vi "Double FFT Mesurament RT (with BackNoise Remove) with Frequency Linearization Test.vi"() -> ()   [LabVIEW 2014]
uses:
  <vilib>/Platform/TimedLoop/XDataNode/timing_clust.ctl
  <vilib>/Platform/TimedLoop/XDataNode/nitl_modes.ctl
  <vilib>/Platform/TimedLoop/XDataNode/wakeup.ctl
  <vilib>/FPGAPlugInAG/sbRIO-9636/niLvFpga_Open_sbRIO-9636.vi
  <vilib>/rvi/interface/common/dynamic/niFpgaDynamicAddResources.vi
  <vilib>/Utility/error.llb/Error Cluster From Error Code.vi
  <vilib>/rvi/errors/niLvFpgaAdjustHostInterfaceError.vi
  <vilib>/rvi/interface/common/niFpgaWaitOnOcc.vi
  <vilib>/FPGAPlugInAG/Dynamic/niLvFpga_Run_Dynamic.vi
  <vilib>/FPGAPlugInAG/Dynamic/niLvFpga_Abort_Dynamic.vi
  <vilib>/FPGAPlugInAG/Dynamic/niLvFpga_Reset_Dynamic.vi
  <vilib>/FPGAPlugInAG/Dynamic/niLvFpga_Close_Dynamic.vi
  <vilib>/rvi/interface/nirviOpenFPGA/nirviOpenFPGA.xnode
  FPGA Bitfiles/LaserDistanceSen_FPGATarget_DoubleFFTMesuram_6dDziXQAIGE.lvbitx
  FPGA Target/Test VIs/Double FFT Mesurament Test with Background Noise Remove.vi
  <vilib>/rvi/interface/nirviReadWriteControl/nirviReadWriteControl.xnode
  <vilib>/rvi/interface/nirviMethod/nirviMethod.xnode
  <vilib>/Platform/TimedLoop/XDataNode/XDataNode.xnode
  <vilib>/rvi/interface/nirviCloseFPGA/nirviCloseFPGA.xnode
  <vilib>/FPGAPlugInAG/Dynamic/niLvFpga_ConfigureFifo_Dynamic.vi
  <vilib>/rvi/errors/niLvFpgaMergeErrorWithErrorCode.vi
  <vilib>/FPGAPlugInAG/Dynamic/niLvFpga_StartFifo_Dynamic.vi
  <vilib>/rvi/interface/Simulation/niFpgaSimulationCallBeginRW.vi
  <vilib>/FPGAPlugInAG/Dynamic/niLvFpga_ReadFifo_Dynamic.vi
  <vilib>/Platform/TimedLoop/XDataNode/XDNodeRunTimeDep.lvlib
  NiFpgaLv.dll
panel:
  in  "SubtractionType":T1(ring)
  out "Fondo Signal":dbl[](graph)
  in  "nbit":i32=7
  in  "LowPass Filter: Low cutoff frequency":dbl=20000.0 format="%#_13g"
  in  "PolyFitting: Poly Grade":dbl=5.0
  in  "Scale Factor Rising":dbl=0.5
  out "2) Std Dev":dbl
  out "1) Std Dev":dbl
  in  "Scale Factor Falling":dbl=0.5
  in  "Triangolo dritto":bool=TRUE
  in  "Acrive  Smooth":bool
  out "Complete SkewTri":dbl[](graph)
  out "2) Tri edge RISING":dbl[](graph)
  out "1) Tri edge FALLING":dbl[](graph)
  out "1) Ext Mean Time Curve":dbl[](graph)
  out "2) Ext Mean Time Curve":dbl[](graph)
  out "2) Mean Freq Curve Rising":dbl[](graph)
  out "1) Mean Freq Curve Falling":dbl[](graph)
  out "2) Freq curve":dbl[](graph)
  out "1) Freq curve":dbl[](graph)
  in  "FFT Sliding Win Size":i32=128
  out "1) SmoothSubSig":dbl[](graph)
  out "2) SmoothSubSig":dbl[](graph)
  in  "Acrive Fit":bool=TRUE
  in  "Poly Order":i32=3
  in  "Side points":i32=13
  in  "Poly Grade":dbl=5.0
  out "2) Signal&Fit 2":dbl[][](graph)
  out "1) Signal&Fit":dbl[][](graph)
  in  "tieni premuto per":i32=1
  out "Current Sig lin":i32
  in  "Acrive Linearization":bool
  in  "# Measurements for Linearization":i32=10
  in  "?":bool
  out "maxbin_secondFFT":i32
  out "maxbin_firstFFT":i32
  out "f_rise":dbl
  out "f_fall":dbl
  out "f_mean":dbl
  out "Velocity (m/s)":dbl
  out "Distance (m)":dbl
  in  "Initial Latency points":u32(slide) scale=0.0..1249.0
  out "Second FFT (bin)":dbl[](graph)
  out "Second Signal (points) - Rising Triangular":dbl[](graph)
  out "First FFT (bin)":dbl[](graph)
  out "First Signal (points) - Falling Triangular":dbl[](graph)
  in  "Snapshot":bool
  in  "Windowing":T2(ring)
  in  "first bin":i32=5
  in  "last bin":i32=255
  in  "lower limit 2":u32(slide)=738 scale=625.0..738.0
  in  "lower limit 1":u32(slide)=113 scale=0.0..113.0
  # "Fondo pre-elaborato"
  # "WARNING:\nOnce pressed wait untill the end of operation"
  # "OFFLINE parameters"
  # "Triangolo storto\nda costante"
  # "Max Detection FFT bin range"
  # "ONLINE parameters"
  # "Se la sottrazione del fondo non è eseguita su FPGA.\n Attivarla per eseguirla lato RT"
  # "Smoothing (S-G Params)"
  # "Fitting"
  # "ONLY POWER OF 2"
  # "Min: 2 Max: 256 (2, 4, 8, 16, 32, 64, 128, 256)"
  # "LINEARIZATION FINAL RESULTS"
  # "dev standard (max-min)"
  # "%"
  # "%"
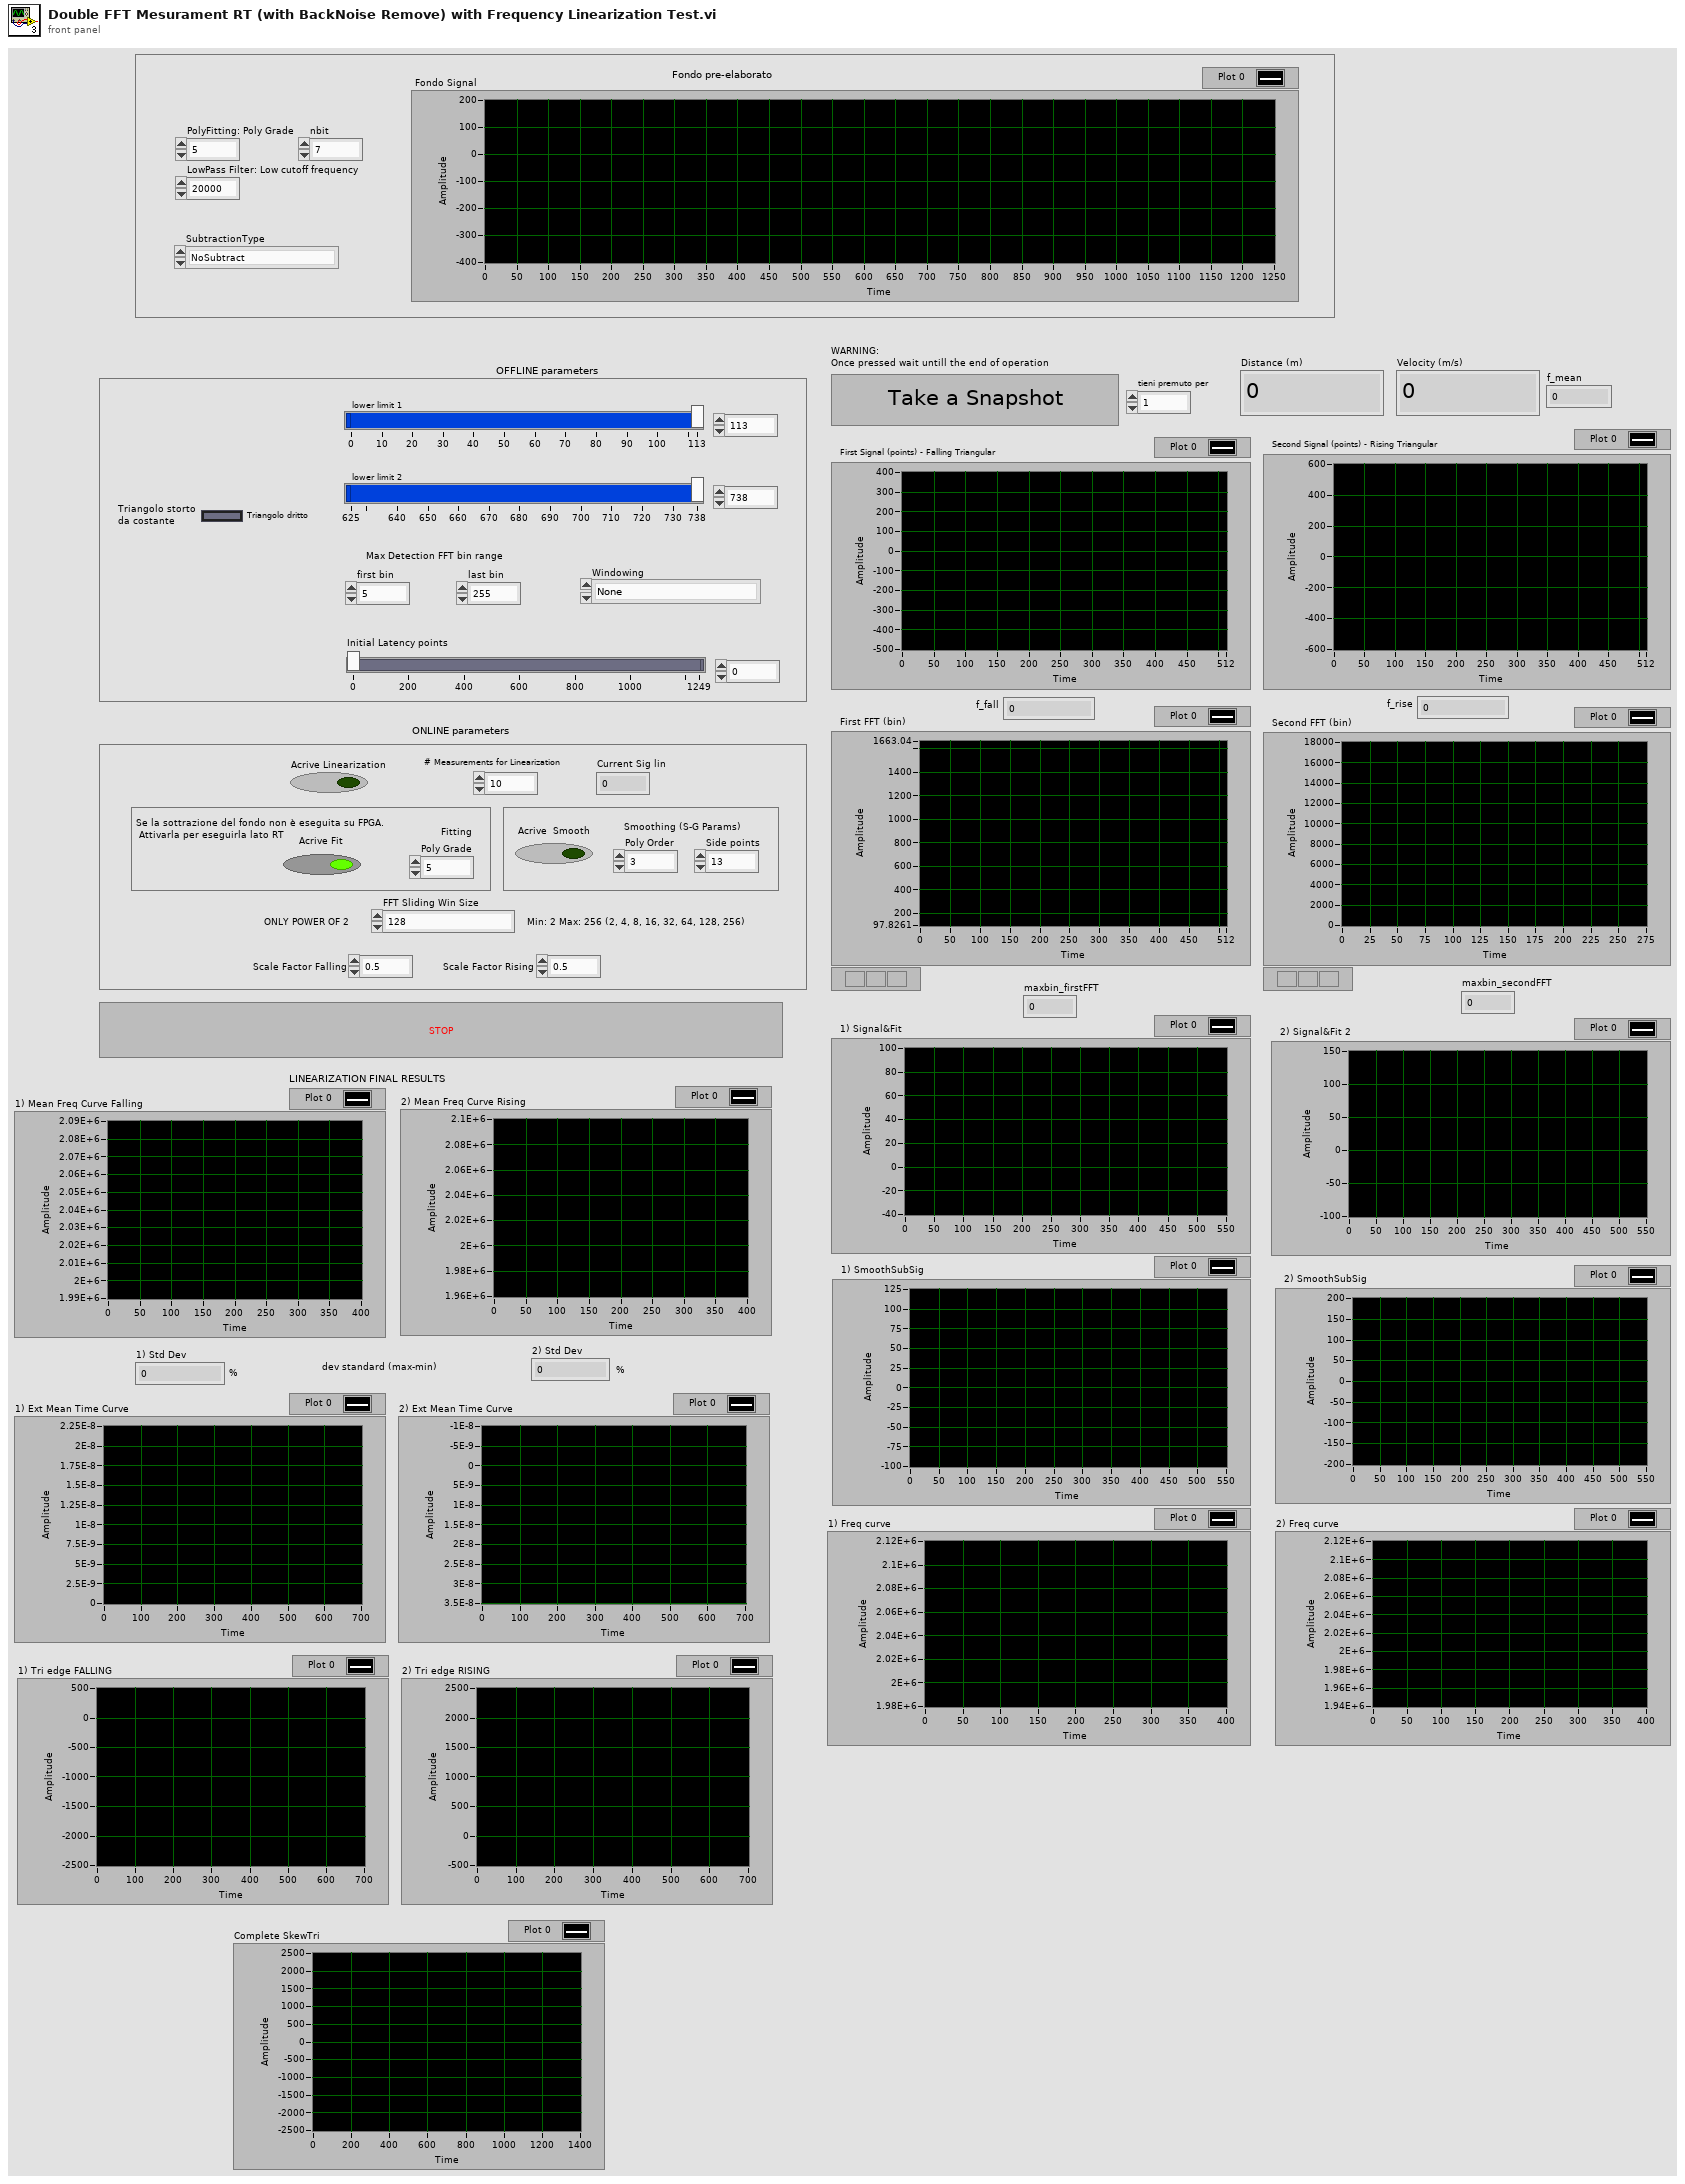
[diagram p1: front panel]
types:
  T1 = enum16{"NoSubtract", "StartingCurve", "LowPass", "PolyFitting"}
  T2 = enum16{"None", "Hanning", "Hamming", "Blackman", "Blackman-Harris"}
  T3 = typedef "XDNodeRunTimeDep.lvlib/timing_clust.ctl" = cluster{"Expected End [f-1]":u64, "Actual End [f-1]":u64, "Finished Late? [f-1]":bool, "Expected End [i-1]":u64, "Actual End [i-1]":u64, "Finished Late? [i-1]":bool, "Expected Start [i]":u64, "Actual Start [i]":u64, "Expected Start [f]":u64, "Actual Start [f]":u64, "Source Name":string, "Structure Name":string, "Period":i64, "Deadline":i64, "Offset":i64, "Start":i64, "Priority":i32, "Timeout":i32, "Mode":T4, "Wakeup Reason":T5, "Error":errorcluster, "Source Type":string, "Secondary Source Type":string, "Global End Time":u64, "Global Start Time":u64, "Frame Duration":u64, "Iteration Duration":u64, "Assigned CPU":i32, "I/O Scan Engine Mode":u32}
  T4 = typedef "XDNodeRunTimeDep.lvlib/nitl_modes.ctl" = enum32{"No Change", "Process missed periods, maintain original phase", "Discard missed periods, maintain original phase", "Process missed periods, ignore original phase", "Discard missed periods, ignore original phase"}
  T5 = typedef "XDNodeRunTimeDep.lvlib/wakeup.ctl" = enum32{"Normal", "Aborted", "Asynchronous wakeup", "Timing source error", "Timed loop error", "Timeout"}
  T6 = typedef "NI_Matrix.lvlib/RealMatrix.ctl" = dbl[][]
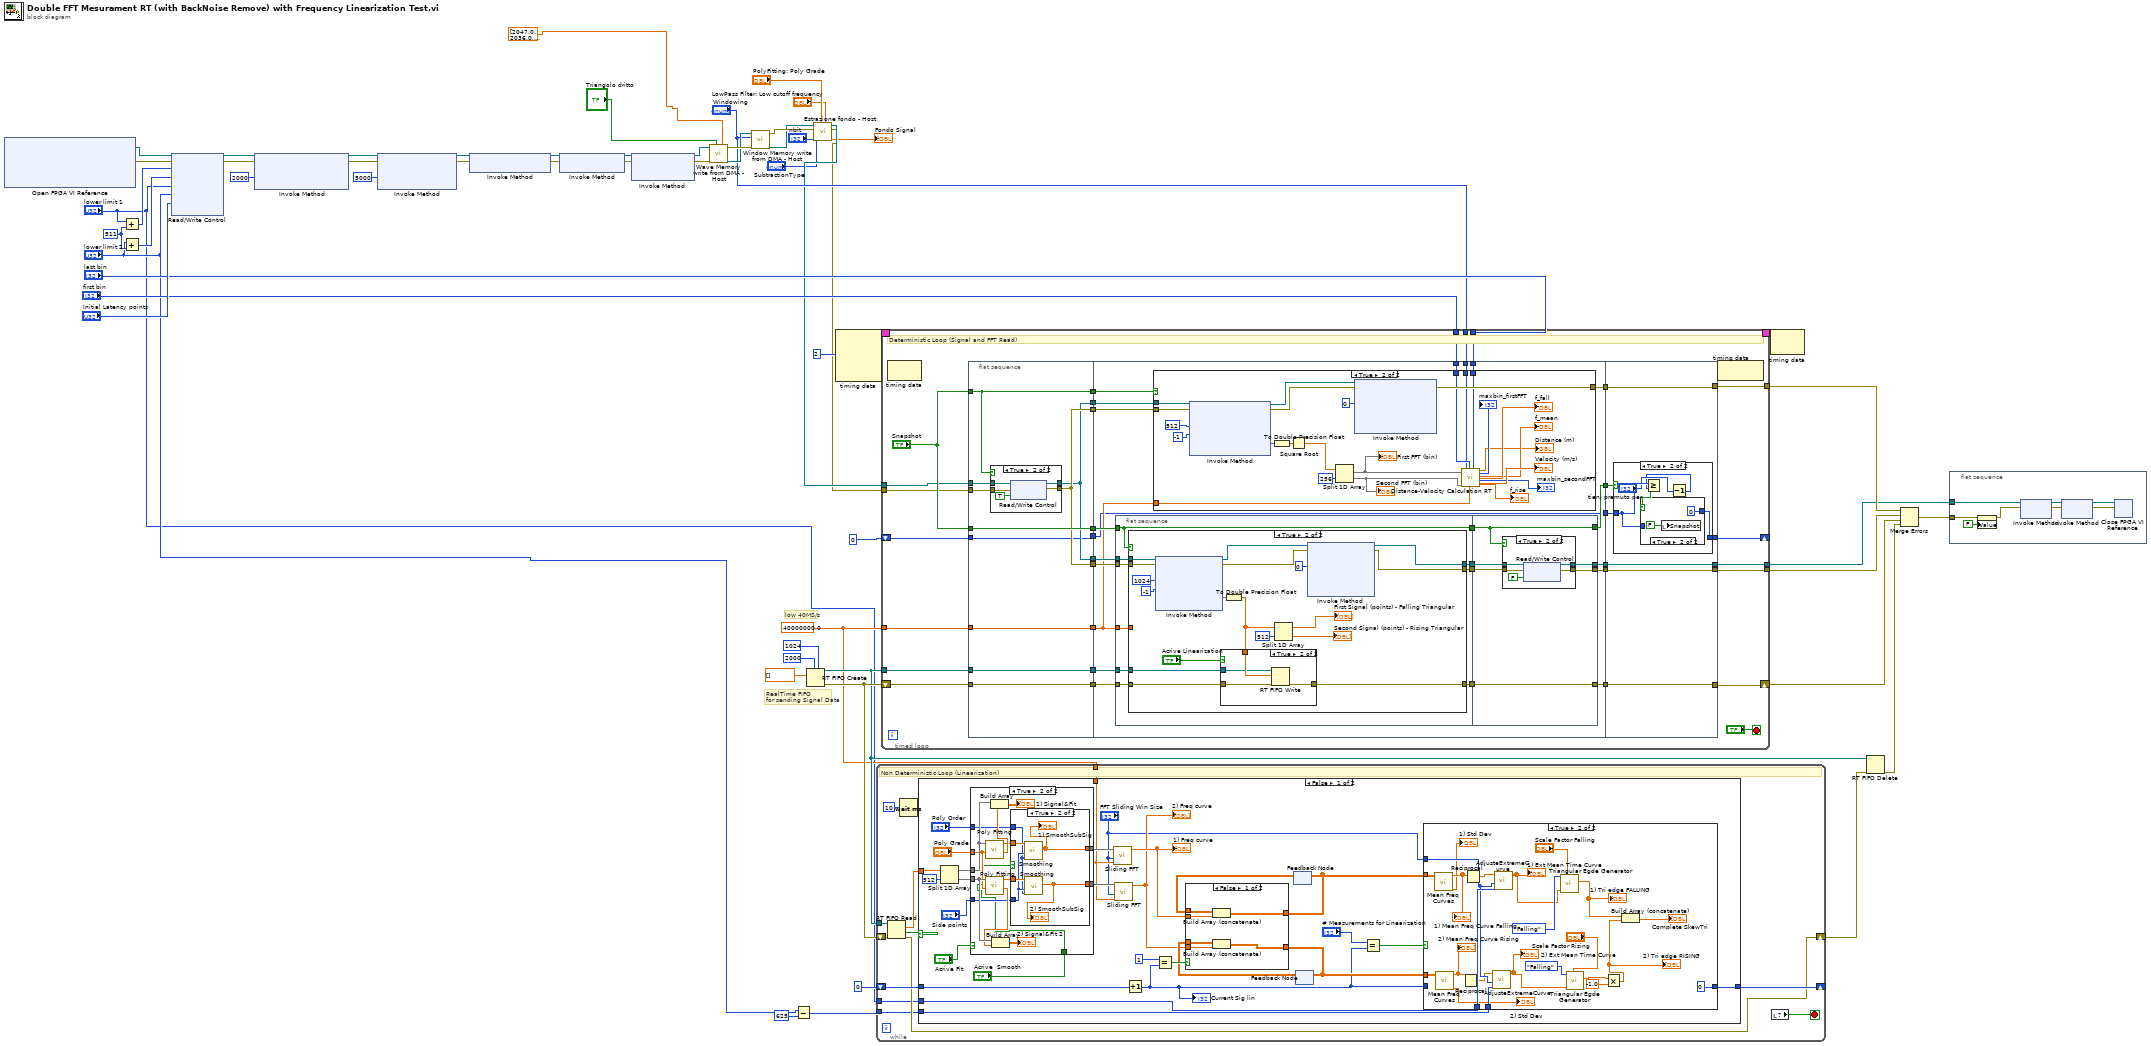
[diagram p0: block diagram]
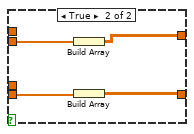
[diagram p5: hidden frame]
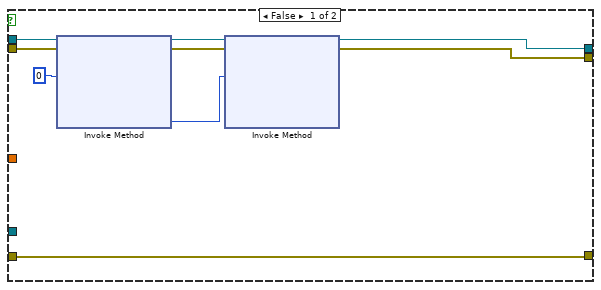
[diagram p8: hidden frame]
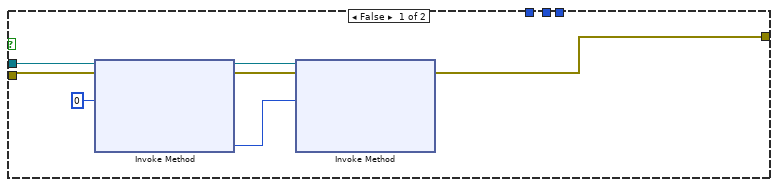
[diagram p11: hidden frame]
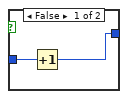
[diagram p13: hidden frame]
diagram:
  w56 = u32 511 ("y")
  w13 = 40000000.0 ("Sample Rate (S/s)")
  # "RealTime FIFO \nfor sending Signal Data"
  # "low 40MS/s"
  n1 = xnode "Open FPGA VI Reference"() -> ("FPGA VI Reference Out"=w55:refnum<k20>, "error out"=w54:errorcluster)  [unwired: 2 in]
  n2 = Add(x="lower limit 1", y=w56) -> (x+y=w58:u32)
  n3 = Add(x="lower limit 2", y=w56) -> (x+y=w57:u32)
  n4 = xnode "Read/Write Control"("FPGA VI Reference In"=w55, "error in"=w54, "upper limit 1"=w58, "upper limit 2"=w57, "lower limit 1"="lower limit 1", "lower limit 2"="lower limit 2", "Latency points"="Initial Latency points") -> ("FPGA VI Reference Out"=w53:refnum<k20>, "error out"=w52:errorcluster)  [unwired: 1 in]
  n5 = xnode "Invoke Method"("FPGA VI Reference In"=w53, "error in"=w52, "Requested Depth"=u32 2000) -> ("FPGA VI Reference Out"=w31:refnum<k20>, "error out"=w32:errorcluster)  [unwired: 1 out]
  n6 = xnode "Invoke Method"("FPGA VI Reference In"=w31, "error in"=w32, "Requested Depth"=u32 5000) -> ("FPGA VI Reference Out"=w45:refnum<k20>, "error out"=w46:errorcluster)  [unwired: 1 out]
  n7 = xnode "Invoke Method"("FPGA VI Reference In"=w45, "error in"=w46) -> ("FPGA VI Reference Out"=w29:refnum<k20>, "error out"=w30:errorcluster)
  n8 = xnode "Invoke Method"("FPGA VI Reference In"=w29, "error in"=w30) -> ("FPGA VI Reference Out"=w43:refnum<k20>, "error out"=w44:errorcluster)
  n9 = xnode "Invoke Method"("FPGA VI Reference In"=w43, "error in"=w44) -> ("FPGA VI Reference Out"=w49:refnum<k20>, "error out"=w48:errorcluster)  [unwired: 1 in]
  n10 = call "Wave Memory write from DMA - Host.vi"("Custom Triangular Signal (fal-ris)"=dbl[] [2047.0, 2036.0, 2024.0, 2013.0, 2002.0, 1990.0, 1979.0, 1968.0, 1956.0, 1945.0, 1934.0, 1923.0, 1912.0, 1900.0, 1889.0, 1878.0, 1867.0, 1856.0, 1845.0, 1833.0, 1822.0, 1811.0, 1800.0, 1789.0, 1778.0, 1767.0, 1756.0, 1745.0, 1734.0, 1723.0, 1712.0, 1702.0, 1691.0, 1680.0, 1669.0, 1658.0, 1647.0, 1636.0, 1626.0, 1615.0, 1604.0, 1593.0, 1583.0, 1572.0, 1561.0, 1550.0, 1540.0, 1529.0, 1518.0, 1508.0, 1497.0, 1487.0, 1476.0, 1465.0, 1455.0, 1444.0, 1434.0, 1423.0, 1413.0, 1402.0, 1392.0, 1381.0, 1371.0, 1360.0, 1350.0, 1340.0, 1329.0, 1319.0, 1309.0, 1298.0, 1288.0, 1278.0, 1267.0, 1257.0, 1247.0, 1237.0, 1226.0, 1216.0, 1206.0, 1196.0, 1186.0, 1176.0, 1165.0, 1155.0, 1145.0, 1135.0, 1125.0, 1115.0, 1105.0, 1095.0, 1085.0, 1075.0, 1065.0, 1055.0, 1045.0, 1035.0, 1025.0, 1015.0, 1006.0, 996.0, 986.0, 976.0, 966.0, 956.0, 947.0, 937.0, 927.0, 917.0, 908.0, 898.0, 888.0, 879.0, 869.0, 859.0, 850.0, 837.0, 826.0, 816.0, 804.0, 796.0, 788.0, 778.0, 769.0, 758.0, 750.0, 743.0, 733.0, 724.0, 717.0, 709.0, 701.0, 693.0, 686.0, 677.0, 669.0, 661.0, 653.0, 645.0, 638.0, 630.0, 622.0, 615.0, 607.0, 599.0, 592.0, 583.0, 576.0, 569.0, 561.0, 554.0, 547.0, 539.0, 532.0, 525.0, 518.0, 509.0, 501.0, 492.0, 486.0, 478.0, 471.0, 463.0, 456.0, 450.0, 442.0, 435.0, 429.0, 421.0, 415.0, 408.0, 401.0, 394.0, 388.0, 381.0, 375.0, 368.0, 361.0, 355.0, 349.0, 342.0, 336.0, 330.0, 323.0, 317.0, 311.0, 304.0, 298.0, 292.0, 286.0, 279.0, 273.0, 267.0, 261.0, 255.0, 249.0, 242.0, 236.0, 230.0, 224.0, 218.0, 212.0, 206.0, 200.0, 194.0, 187.0, 181.0, 175.0, 169.0, 163.0, 157.0, 150.0, 144.0, 138.0, 132.0, 125.0, 119.0, 113.0, 107.0, 101.0, 95.0, 88.0, 82.0, 77.0, 71.0, 65.0, 59.0, 53.0, 47.0, 41.0, 35.0, 29.0, 23.0, 18.0, 11.0, 6.0, 0.0, -6.0, -12.0, -18.0, -23.0, -29.0, -35.0, -41.0, -47.0, -52.0, -58.0, -64.0, -69.0, -75.0, -81.0, -87.0, -92.0, -98.0, -104.0, -109.0, -115.0, -121.0, -126.0, -132.0, -138.0, -144.0, -149.0, -155.0, -161.0, -166.0, -172.0, -177.0, -183.0, -189.0, -194.0, -200.0, -205.0, -211.0, -216.0, -222.0, -227.0, -233.0, -238.0, -244.0, -249.0, -255.0, -260.0, -266.0, -271.0, -277.0, -283.0, -288.0, -294.0, -299.0, -304.0, -310.0, -315.0, -321.0, -326.0, -331.0, -337.0, -342.0, -348.0, -353.0, -358.0, -364.0, -369.0, -375.0, -380.0, -385.0, -391.0, -396.0, -402.0, -407.0, -413.0, -418.0, -423.0, -429.0, -434.0, -439.0, -445.0, -450.0, -456.0, -461.0, -466.0, -472.0, -477.0, -483.0, -488.0, -493.0, -499.0, -504.0, -510.0, -515.0, -520.0, -526.0, -531.0, -537.0, -542.0, -548.0, -553.0, -558.0, -564.0, -569.0, -574.0, -580.0, -585.0, -590.0, -596.0, -601.0, -606.0, -612.0, -617.0, -622.0, -628.0, -633.0, -638.0, -644.0, -649.0, -654.0, -660.0, -665.0, -670.0, -676.0, -681.0, -686.0, -692.0, -697.0, -702.0, -708.0, -713.0, -718.0, -723.0, -729.0, -734.0, -739.0, -744.0, -750.0, -755.0, -760.0, -765.0, -771.0, -776.0, -781.0, -786.0, -792.0, -797.0, -802.0, -807.0, -812.0, -818.0, -823.0, -828.0, -833.0, -839.0, -844.0, -849.0, -854.0, -859.0, -865.0, -870.0, -875.0, -880.0, -885.0, -891.0, -896.0, -901.0, -906.0, -911.0, -916.0, -922.0, -927.0, -932.0, -937.0, -943.0, -948.0, -953.0, -958.0, -963.0, -969.0, -974.0, -979.0, -984.0, -989.0, -995.0, -1000.0, -1005.0, -1010.0, -1015.0, -1021.0, -1026.0, -1031.0, -1036.0, -1041.0, -1047.0, -1052.0, -1057.0, -1062.0, -1067.0, -1073.0, -1078.0, -1083.0, -1088.0, -1093.0, -1099.0, -1104.0, -1109.0, -1114.0, -1119.0, -1124.0, -1130.0, -1135.0, -1140.0, -1145.0, -1150.0, -1156.0, -1161.0, -1166.0, -1171.0, -1176.0, -1182.0, -1187.0, -1192.0, -1197.0, -1202.0, -1207.0, -1213.0, -1218.0, -1223.0, -1228.0, -1233.0, -1238.0, -1244.0, -1249.0, -1254.0, -1259.0, -1264.0, -1269.0, -1275.0, -1280.0, -1285.0, -1290.0, -1295.0, -1300.0, -1305.0, -1311.0, -1316.0, -1321.0, -1326.0, -1331.0, -1336.0, -1342.0, -1347.0, -1352.0, -1357.0, -1362.0, -1367.0, -1372.0, -1378.0, -1383.0, -1388.0, -1393.0, -1398.0, -1403.0, -1408.0, -1414.0, -1419.0, -1424.0, -1429.0, -1434.0, -1439.0, -1444.0, -1450.0, -1455.0, -1460.0, -1465.0, -1470.0, -1475.0, -1480.0, -1486.0, -1491.0, -1496.0, -1501.0, -1506.0, -1511.0, -1516.0, -1522.0, -1527.0, -1532.0, -1537.0, -1542.0, -1547.0, -1552.0, -1558.0, -1563.0, -1568.0, -1573.0, -1578.0, -1583.0, -1588.0, -1593.0, -1599.0, -1604.0, -1609.0, -1614.0, -1619.0, -1624.0, -1629.0, -1634.0, -1640.0, -1645.0, -1650.0, -1655.0, -1660.0, -1665.0, -1670.0, -1675.0, -1681.0, -1686.0, -1691.0, -1696.0, -1701.0, -1706.0, -1711.0, -1716.0, -1722.0, -1727.0, -1732.0, -1737.0, -1742.0, -1747.0, -1752.0, -1757.0, -1762.0, -1768.0, -1773.0, -1778.0, -1783.0, -1788.0, -1793.0, -1798.0, -1803.0, -1808.0, -1814.0, -1819.0, -1824.0, -1829.0, -1834.0, -1839.0, -1844.0, -1849.0, -1854.0, -1859.0, -1865.0, -1870.0, -1875.0, -1880.0, -1885.0, -1890.0, -1895.0, -1900.0, -1905.0, -1911.0, -1916.0, -1921.0, -1926.0, -1931.0, -1936.0, -1941.0, -1946.0, -1951.0, -1956.0, -1961.0, -1967.0, -1972.0, -1977.0, -1982.0, -1987.0, -1992.0, -1997.0, -2002.0, -2007.0, -2012.0, -2017.0, -2023.0, -2028.0, -2033.0, -2038.0, -2043.0, -2048.0, -2047.0, -2034.0, -2021.0, -2009.0, -1996.0, -1983.0, -1970.0, -1957.0, -1945.0, -1932.0, -1919.0, -1907.0, -1894.0, -1881.0, -1869.0, -1856.0, -1844.0, -1831.0, -1819.0, -1806.0, -1794.0, -1781.0, -1769.0, -1757.0, -1744.0, -1732.0, -1719.0, -1707.0, -1695.0, -1682.0, -1670.0, -1658.0, -1646.0, -1634.0, -1621.0, -1609.0, -1597.0, -1585.0, -1573.0, -1561.0, -1549.0, -1537.0, -1525.0, -1513.0, -1501.0, -1489.0, -1477.0, -1465.0, -1453.0, -1441.0, -1429.0, -1417.0, -1405.0, -1394.0, -1382.0, -1370.0, -1358.0, -1347.0, -1335.0, -1323.0, -1312.0, -1300.0, -1288.0, -1277.0, -1265.0, -1254.0, -1242.0, -1231.0, -1219.0, -1208.0, -1196.0, -1185.0, -1173.0, -1162.0, -1150.0, -1139.0, -1128.0, -1116.0, -1105.0, -1094.0, -1083.0, -1071.0, -1060.0, -1049.0, -1038.0, -1027.0, -1015.0, -1004.0, -993.0, -982.0, -971.0, -960.0, -949.0, -938.0, -927.0, -916.0, -905.0, -894.0, -883.0, -873.0, -862.0, -851.0, -840.0, -829.0, -819.0, -808.0, -797.0, -786.0, -776.0, -765.0, -754.0, -744.0, -733.0, -722.0, -712.0, -697.0, -685.0, -674.0, -661.0, -652.0, -643.0, -632.0, -622.0, -610.0, -602.0, -594.0, -583.0, -574.0, -566.0, -558.0, -550.0, -542.0, -534.0, -525.0, -516.0, -507.0, -499.0, -491.0, -483.0, -475.0, -467.0, -459.0, -451.0, -443.0, -435.0, -426.0, -419.0, -411.0, -404.0, -396.0, -388.0, -381.0, -373.0, -366.0, -359.0, -349.0, -341.0, -331.0, -325.0, -317.0, -309.0, -301.0, -295.0, -288.0, -280.0, -273.0, -266.0, -259.0, -252.0, -246.0, -239.0, -231.0, -225.0, -219.0, -212.0, -205.0, -199.0, -192.0, -186.0, -180.0, -173.0, -167.0, -161.0, -155.0, -148.0, -142.0, -136.0, -130.0, -124.0, -118.0, -112.0, -106.0, -100.0, -94.0, -88.0, -82.0, -76.0, -70.0, -64.0, -58.0, -52.0, -46.0, -40.0, -34.0, -28.0, -21.0, -15.0, -9.0, -3.0, 2.0, 9.0, 15.0, 21.0, 27.0, 33.0, 39.0, 45.0, 51.0, 57.0, 63.0, 69.0, 75.0, 81.0, 86.0, 92.0, 98.0, 103.0, 110.0, 116.0, 121.0, 127.0, 133.0, 138.0, 144.0, 149.0, 155.0, 161.0, 166.0, 172.0, 177.0, 183.0, 189.0, 194.0, 200.0, 205.0, 211.0, 216.0, 221.0, 227.0, 232.0, 238.0, 243.0, 249.0, 254.0, 259.0, 265.0, 270.0, 276.0, 281.0, 286.0, 292.0, 297.0, 303.0, 308.0, 314.0, 319.0, 324.0, 329.0, 335.0, 340.0, 345.0, 351.0, 356.0, 361.0, 366.0, 371.0, 377.0, 382.0, 387.0, 392.0, 397.0, 403.0, 408.0, 413.0, 418.0, 423.0, 429.0, 434.0, 439.0, 444.0, 449.0, 454.0, 459.0, 464.0, 469.0, 474.0, 479.0, 484.0, 489.0, 494.0, 499.0, 504.0, 509.0, 514.0, 520.0, 525.0, 530.0, 535.0, 540.0, 545.0, 550.0, 555.0, 560.0, 565.0, 570.0, 575.0, 580.0, 585.0, 590.0, 595.0, 600.0, 605.0, 610.0, 615.0, 620.0, 625.0, 630.0, 636.0, 641.0, 646.0, 651.0, 656.0, 661.0, 666.0, 671.0, 676.0, 681.0, 686.0, 691.0, 696.0, 701.0, 706.0, 711.0, 716.0, 721.0, 726.0, 731.0, 736.0, 741.0, 746.0, 751.0, 756.0, 761.0, 765.0, 770.0, 775.0, 780.0, 785.0, 790.0, 795.0, 800.0, 805.0, 810.0, 815.0, 820.0, 825.0, 829.0, 834.0, 839.0, 844.0, 849.0, 854.0, 859.0, 864.0, 868.0, 873.0, 878.0, 883.0, 888.0, 893.0, 897.0, 902.0, 907.0, 912.0, 917.0, 921.0, 926.0, 931.0, 936.0, 941.0, 945.0, 950.0, 955.0, 960.0, 965.0, 969.0, 974.0, 979.0, 984.0, 988.0, 993.0, 998.0, 1003.0, 1007.0, 1012.0, 1017.0, 1022.0, 1027.0, 1031.0, 1036.0, 1041.0, 1046.0, 1051.0, 1055.0, 1060.0, 1065.0, 1070.0, 1075.0, 1079.0, 1084.0, 1089.0, 1094.0, 1098.0, 1103.0, 1108.0, 1113.0, 1118.0, 1122.0, 1127.0, 1132.0, 1137.0, 1141.0, 1146.0, 1151.0, 1156.0, 1161.0, 1165.0, 1170.0, 1175.0, 1180.0, 1184.0, 1189.0, 1194.0, 1199.0, 1204.0, 1208.0, 1213.0, 1218.0, 1223.0, 1227.0, 1232.0, 1237.0, 1242.0, 1246.0, 1251.0, 1256.0, 1261.0, 1265.0, 1270.0, 1275.0, 1280.0, 1284.0, 1289.0, 1294.0, 1299.0, 1303.0, 1308.0, 1313.0, 1318.0, 1322.0, 1327.0, 1332.0, 1336.0, 1341.0, 1346.0, 1351.0, 1355.0, 1360.0, 1365.0, 1370.0, 1374.0, 1379.0, 1384.0, 1388.0, 1393.0, 1398.0, 1403.0, 1407.0, 1412.0, 1417.0, 1421.0, 1426.0, 1431.0, 1436.0, 1440.0, 1445.0, 1450.0, 1454.0, 1459.0, 1464.0, 1469.0, 1473.0, 1478.0, 1483.0, 1487.0, 1492.0, 1497.0, 1502.0, 1506.0, 1511.0, 1516.0, 1520.0, 1525.0, 1530.0, 1535.0, 1539.0, 1544.0, 1549.0, 1553.0, 1558.0, 1563.0, 1567.0, 1572.0, 1577.0, 1582.0, 1586.0, 1591.0, 1596.0, 1600.0, 1605.0, 1610.0, 1614.0, 1619.0, 1624.0, 1628.0, 1633.0, 1638.0, 1643.0, 1647.0, 1652.0, 1657.0, 1661.0, 1666.0, 1671.0, 1675.0, 1680.0, 1685.0, 1689.0, 1694.0, 1699.0, 1703.0, 1708.0, 1713.0, 1717.0, 1722.0, 1727.0, 1731.0, 1736.0, 1741.0, 1746.0, 1750.0, 1755.0, 1760.0, 1764.0, 1769.0, 1774.0, 1778.0, 1783.0, 1788.0, 1792.0, 1797.0, 1802.0, 1806.0, 1811.0, 1816.0, 1820.0, 1825.0, 1830.0, 1834.0, 1839.0, 1844.0, 1848.0, 1853.0, 1858.0, 1862.0, 1867.0, 1871.0, 1876.0, 1881.0, 1885.0, 1890.0, 1895.0, 1899.0, 1904.0, 1909.0, 1913.0, 1918.0, 1923.0, 1927.0, 1932.0, 1937.0, 1941.0, 1946.0, 1951.0, 1955.0, 1960.0, 1965.0, 1969.0, 1974.0, 1978.0, 1983.0, 1988.0, 1992.0, 1997.0, 2002.0, 2006.0, 2011.0, 2016.0, 2020.0, 2025.0, 2029.0, 2034.0, 2039.0, 2043.0, 2048.0] ("Complete SkewTri"), "Triangolo dritto?"="Triangolo dritto", "error in"=w48, "FPGA VI Reference In"=w49) -> ("FPGA VI Reference Out"=w34:refnum<k20>, "error out"=w47:errorcluster)  [unwired: 5 in, 1 out]
  n11 = call "Window Memory write from DMA - Host.vi"("error in"=w47, "Enum"="Windowing", "FPGA VI Reference In"=w34) -> ("FPGA VI Reference Out"=w8:refnum<k20>, "error out"=w9:errorcluster)  [unwired: 5 in, 2 out]
  n12 = Subtract(x="lower limit 2", y=u32 625) -> (x-y=w15:u32)
  n13 = RT FIFO Create(1:dbl[] [] ("double precision float"), 4:u32 2000 ("size (10)"), 6:u32 1024 ("elements in array (1)")) -> (8:w21:refnum<k33>, 11:w23:errorcluster)  [unwired: 5 in, 1 out]
  n14 = call "Estrazione fondo - Host.vi"("LowPass Filter: Low cutoff frequency"="LowPass Filter: Low cutoff frequency", "PolyFitting: Poly Grade"="PolyFitting: Poly Grade", "nbit"="nbit", "SubtractionType"="SubtractionType", "error in"=w9, "FPGA VI Reference In"=w8) -> ("Fondo Signal"=→"Fondo Signal":dbl[], "error out"=w6:errorcluster, "FPGA VI Reference Out"=w7:refnum<k20>)  [unwired: 2 in, 1 out]
  n15 = node-c288(i64 2 ("Period")) -> (w42:T3)  [unwired: 3 in]
  n16 = while {
    shift-right: [w62] -> w20
    shift-left: w23 -> [w64]
    tunnel: w21 -> [w69]
    shift-right: [w63] -> _
    shift-left: 0 -> [w67]
    tunnel: "lower limit 1" -> [w59]
    tunnel: w15 -> [w60]
    tunnel: w13 -> [w61]
    stop <- w68 stop-if-true
    # "Non Deterministic Loop (Linearization)"
    n17 = RT FIFO Read(0:w69, 3:w64) -> (9:w66:dbl[], 10:w65:bool, 11:w62:errorcluster)  [unwired: 2 in, 2 out]
    n18 = Wait (ms)(milliseconds to wait=u32 10 ("millisecond multiple")) -> ()  [unwired: 1 out]
    n19 = case shown="False" w65 {
      tunnel: w67 -> [w98 w157]
      tunnel: [w87 w157] -> w63
      tunnel: w66 -> [w96 _]
      tunnel: w61 -> [w77 _]
      tunnel: w60 -> [w74 _]
      tunnel: w59 -> [w73 _]
      frame False {
        n20 = Split 1D Array(array=w96, index=512) -> (first subarray=w85:dbl[], second subarray=w84:dbl[])
        n21 = case shown="True" "Acrive Fit" {
          tunnel: w85 -> [w100 w114]
          tunnel: w84 -> [w99 w110]
          tunnel: "Poly Grade" -> [_ w106]
          tunnel: "Side points" -> [_ w105]
          tunnel: "Poly Order" -> [_ w104]
          tunnel: [w99 w103] -> w78
          tunnel: [w100 w101] -> w79
          tunnel: "Acrive  Smooth" -> [_ w102]
          frame False {
          }
          frame True {
            n22 = call "Poly Fitting.vi"("Poly Grade"=w106, "Signal"=w114) -> ("Poly Signal"=w113:dbl[], "SubtractedSignal"=w108:dbl[])  [unwired: 8 in]
            n23 = call "Poly Fitting.vi"("Poly Grade"=w106, "Signal"=w110) -> ("Poly Signal"=w109:dbl[], "SubtractedSignal"=w107:dbl[])  [unwired: 8 in]
            n24 = Build Array(w114, w113) -> (→"1) Signal&Fit":dbl[][])
            n25 = Build Array(w110, w109) -> (→"2) Signal&Fit 2":dbl[][])
            n26 = case shown="True" w102 {
              tunnel: w108 -> [w116 w122]
              tunnel: w107 -> [w115 w121]
              tunnel: w105 -> [_ w120]
              tunnel: w104 -> [_ w119]
              tunnel: [w115 w118] -> w103
              tunnel: [w116 w117] -> w101
              frame False {
              }
              frame True {
                n27 = call "Smoothing.vi"("polynomial order"=w119, "side points"=w120, "SubtractedSignal"=w122) -> ("SubSmoothSignal"=w117:dbl[])  [unwired: 8 in]
                "1) SmoothSubSig" <- w117
                n28 = call "Smoothing.vi"("polynomial order"=w119, "side points"=w120, "SubtractedSignal"=w121) -> ("SubSmoothSignal"=w118:dbl[])  [unwired: 8 in]
                "2) SmoothSubSig" <- w118
              }
            }
          }
        }
        n29 = call "Sliding FFT.vi"("Sample Freq"=w77, "FFT Win Size"="FFT Sliding Win Size", "SubSmoothSignal"=w79) -> ("Freq samples"=w76:dbl[])  [unwired: 7 in, 1 out]
        "1) Freq curve" <- w76
        n30 = call "Sliding FFT.vi"("Sample Freq"=w77, "FFT Win Size"="FFT Sliding Win Size", "SubSmoothSignal"=w78) -> ("Freq samples"=w75:dbl[])  [unwired: 7 in, 1 out]
        "2) Freq curve" <- w75
        n31 = Increment(x=w98) -> (x+1=w88:i32)
        "Current Sig lin" <- w88
        n32 = Equal?(x=1, y=w88) -> (x = y?=w94:bool)
        n33 = feedback #1() -> (w93:T6)  [unwired: 1 in]
        n34 = feedback #2() -> (w92:T6)  [unwired: 1 in]
        n35 = case shown="False" w94 {
          tunnel: w75 -> [w151 w154]
          tunnel: w76 -> [w152 w156]
          tunnel: [w150 w153] -> w89
          tunnel: [w149 w155] -> w90
          tunnel: w93 -> [w148 _]
          tunnel: w92 -> [w147 _]
          frame False {
            n36 = Build Array (concatenate)(w148, w152) -> (w149:T6)
            n37 = Build Array (concatenate)(w147, w151) -> (w150:T6)
          }
          frame True {
            n38 = Build Array(w156) -> (w155:T6)
            n39 = Build Array(w154) -> (w153:T6)
          }
        }
        n40 = feedback-in #1(w90) -> ()
        n41 = feedback-in #2(w89) -> ()
        n42 = Equal?(x="# Measurements for Linearization", y=w88) -> (x = y?=w86:bool)
        n43 = case shown="True" w86 {
          tunnel: w90 -> [_ w125]
          tunnel: w89 -> [_ w124]
          tunnel: w88 -> [w123 _]
          tunnel: [w123 0] -> w87
          tunnel: w74 -> [_ w141]
          tunnel: w73 -> [_ w140]
          tunnel: "FFT Sliding Win Size" -> [_ w139]
          frame False {
          }
          frame True {
            n44 = call "Mean Freq Curves.vi"("Set of Freq samples"=w125) -> ("StdDev%"=→"1) Std Dev":dbl, "Mean Freq Curve"=w134:dbl[])  [unwired: 9 in]
            "1) Mean Freq Curve Falling" <- w134
            n45 = call "Mean Freq Curves.vi"("Set of Freq samples"=w124) -> ("StdDev%"=→"2) Std Dev":dbl, "Mean Freq Curve"=w136:dbl[])  [unwired: 9 in]
            "2) Mean Freq Curve Rising" <- w136
            n46 = Reciprocal(x=w136) -> (1/x=w135:dbl[])
            n47 = Reciprocal(x=w134) -> (1/x=w133:dbl[])
            n48 = call "AdjusteExtremeCurve.vi"("Init Bins Discarded"=w141, "FFT Size Window"=w139, "Freq sample"=w135) -> ("Extended Freq Sample"=w137:dbl[])  [unwired: 8 in]
            "2) Ext Mean Time Curve" <- w137
            n49 = call "AdjusteExtremeCurve.vi"("Init Bins Discarded"=w140, "FFT Size Window"=w139, "Freq sample"=w133) -> ("Extended Freq Sample"=w138:dbl[])  [unwired: 8 in]
            "1) Ext Mean Time Curve" <- w138
            n50 = call "Triangular Egde Generator.vi"("fattore"="Scale Factor Falling", "Sample values"=w138, "Triangular edge"=enum16{"Rising", "Falling"}."Falling") -> ("Skew Triangular"=w143:dbl[])  [unwired: 8 in]
            "1) Tri edge FALLING" <- w143
            n51 = call "Triangular Egde Generator.vi"("fattore"="Scale Factor Rising", "Sample values"=w137, "Triangular edge"=enum16{"Rising", "Falling"}."Falling") -> ("Skew Triangular"=w131:dbl[])  [unwired: 8 in]
            n52 = Multiply(x=w131, y=-1.0) -> (x*y=w130:dbl[])
            "2) Tri edge RISING" <- w130
            n53 = Build Array (concatenate)(w143, w130) -> (→"Complete SkewTri":dbl[])
          }
        }
      }
      frame True {
      }
    }
    n54 = local read item#18() -> (w68:bool)
  }
  n55 = timed-loop {
    tunnel: w7 -> [w184]
    tunnel: w6 -> [w185]
    tunnel: [w187] -> w39
    tunnel: w13 -> [w189]
    tunnel: [w188] -> w38
    timing: w42 -> [_]
    timing-out: [_] -> w41
    tunnel: "first bin" -> [w173]
    tunnel: "last bin" -> [w172]
    tunnel: [w170] -> w33
    tunnel: "Windowing" -> [w168]
    shift-right: [w162] -> w24
    shift-left: w23 -> [w164]
    tunnel: w21 -> [w166]
    shift-right: [w158] -> _
    shift-left: 0 -> [w160]
    stop <- "?" stop-if-true
    # "Deterministic Loop (Signal and FFT Read)"
    n56 = node-c288() -> ()  [unwired: 1 in, 1 out]
    n57 = flat-sequence {
      tunnel: w184 -> [w197]
      tunnel: w185 -> [w198]
      tunnel: "Snapshot" -> [w195]
      tunnel: "Snapshot" -> [w200]
      tunnel: w189 -> [w201]
      tunnel: [w199] -> w183
      tunnel: [w201] -> w182
      tunnel: [w200] -> w181
      tunnel: [w195] -> w180
      tunnel: [w199] -> w179
      tunnel: [w196] -> w178
      tunnel: [w196] -> w177
      tunnel: [w194] -> w167
      tunnel: w166 -> [w194]
      tunnel: [w193] -> w165
      tunnel: w164 -> [w193]
      tunnel: [w192] -> w161
      tunnel: w160 -> [w192]
      tunnel: w183 -> [w226]
      tunnel: w182 -> [w214]
      tunnel: w181 -> [w220]
      tunnel: w180 -> [w223]
      tunnel: w179 -> [w222]
      tunnel: w178 -> [w221]
      tunnel: w177 -> [w227]
      tunnel: [w225] -> w176
      tunnel: [w224] -> w175
      tunnel: [w219] -> w174
      tunnel: w173 -> [w218]
      tunnel: w172 -> [w217]
      tunnel: [w216] -> w169
      tunnel: w168 -> [w215]
      tunnel: w167 -> [w213]
      tunnel: w165 -> [w212]
      tunnel: [w210] -> w163
      tunnel: w161 -> [w209]
      tunnel: [w209] -> w159
      tunnel: [w322] -> w187
      tunnel: [w323] -> w188
      tunnel: w176 -> [w323]
      tunnel: w175 -> [w322]
      tunnel: w174 -> [w321]
      tunnel: [w320] -> w170
      tunnel: w169 -> [w320]
      tunnel: [w319] -> w162
      tunnel: w163 -> [w319]
      tunnel: w159 -> [w318]
      tunnel: [w317] -> w158
      frame #0 {
        n58 = case shown="True" w195 {
          tunnel: [w202 w207] -> w199
          tunnel: w198 -> [w202 w206]
          tunnel: w197 -> [w203 w205]
          tunnel: [w203 w204] -> w196
          frame False {
          }
          frame True {
            n59 = xnode "Read/Write Control"("FPGA VI Reference In"=w205, "error in"=w206, "snapshot"=TRUE) -> ("FPGA VI Reference Out"=w204:refnum<k20>, "error out"=w207:errorcluster)
          }
        }
      }
      frame #1 {
        n60 = flat-sequence {
          tunnel: w227 -> [w239]
          tunnel: w226 -> [w238]
          tunnel: w214 -> [w237]
          tunnel: w220 -> [w234]
          tunnel: [w236] -> w230
          tunnel: [w235] -> w229
          tunnel: [w234] -> w228
          tunnel: w213 -> [w233]
          tunnel: w212 -> [w232]
          tunnel: [w231] -> w211
          tunnel: [w275] -> w224
          tunnel: w230 -> [w277]
          tunnel: w229 -> [w276]
          tunnel: w228 -> [w274]
          tunnel: [w274] -> w219
          tunnel: [w273] -> w216
          tunnel: [w272] -> w210
          tunnel: w211 -> [w272]
          frame #0 {
            n61 = case shown="True" w234 {
              tunnel: w239 -> [w247 w266]
              tunnel: w238 -> [w245 w265]
              tunnel: [w244 w258] -> w235
              tunnel: w237 -> [_ _]
              tunnel: [w241 w257] -> w236
              tunnel: w233 -> [_ w252]
              tunnel: w232 -> [w240 w251]
              tunnel: [w240 w250] -> w231
              frame False {
                n62 = xnode "Invoke Method"("FPGA VI Reference In"=w247, "error in"=w245, "Number of Elements"=u32 0) -> ("FPGA VI Reference Out"=w243:refnum<k20>, "error out"=w242:errorcluster, "Elements Remaining"=w246:u32)  [unwired: 1 in, 1 out]
                n63 = xnode "Invoke Method"("FPGA VI Reference In"=w243, "error in"=w242, "Number of Elements"=w246) -> ("FPGA VI Reference Out"=w241:refnum<k20>, "error out"=w244:errorcluster)  [unwired: 1 in, 2 out]
              }
              frame True {
                n64 = xnode "Invoke Method"("FPGA VI Reference In"=w266, "error in"=w265, "Number of Elements"=u32 1024, "Timeout (ms)"=-1) -> ("FPGA VI Reference Out"=w260:refnum<k20>, "error out"=w259:errorcluster, "Data"=w262:fxp<+/-,12,12>[])  [unwired: 1 out]
                n65 = To Double Precision Float(number=w262) -> (double precision float=w253:dbl[])
                n66 = case shown="True" "Acrive Linearization" {
                  tunnel: w253 -> [_ w271]
                  tunnel: w252 -> [_ w270]
                  tunnel: w251 -> [w267 w269]
                  tunnel: [w267 w268] -> w250
                  frame False {
                  }
                  frame True {
                    n67 = RT FIFO Write(0:w270, 1:w271, 3:w269) -> (11:w268:errorcluster)  [unwired: 2 in, 3 out]
                  }
                }
                n68 = Split 1D Array(array=w253, index=512) -> (first subarray=→"First Signal (points) - Falling Triangular":dbl[], second subarray=→"Second Signal (points) - Rising Triangular":dbl[])
                n69 = xnode "Invoke Method"("FPGA VI Reference In"=w260, "error in"=w259, "Number of Elements"=u32 0) -> ("FPGA VI Reference Out"=w257:refnum<k20>, "error out"=w258:errorcluster)  [unwired: 1 in, 2 out]
              }
            }
          }
          frame #1 {
            n70 = case shown="True" w274 {
              tunnel: [w279 w282] -> w275
              tunnel: w277 -> [w278 w283]
              tunnel: w276 -> [w279 w281]
              tunnel: [w278 w280] -> w273
              frame False {
              }
              frame True {
                n71 = xnode "Read/Write Control"("FPGA VI Reference In"=w283, "error in"=w281, "snapshot"=FALSE) -> ("FPGA VI Reference Out"=w280:refnum<k20>, "error out"=w282:errorcluster)
              }
            }
          }
        }
        n72 = case shown="True" w223 {
          tunnel: w221 -> [w290 w311]
          tunnel: w222 -> [w287 w312]
          tunnel: [w286 w310] -> w225
          tunnel: w218 -> [_ w297]
          tunnel: w217 -> [_ w298]
          tunnel: w215 -> [_ w294]
          tunnel: w214 -> [_ w292]
          frame False {
            n73 = xnode "Invoke Method"("FPGA VI Reference In"=w290, "error in"=w287, "Number of Elements"=u32 0) -> ("FPGA VI Reference Out"=w288:refnum<k20>, "error out"=w285:errorcluster, "Elements Remaining"=w289:u32)  [unwired: 1 in, 1 out]
            n74 = xnode "Invoke Method"("FPGA VI Reference In"=w288, "error in"=w285, "Number of Elements"=w289) -> ("error out"=w286:errorcluster)  [unwired: 1 in, 3 out]
          }
          frame True {
            n75 = xnode "Invoke Method"("FPGA VI Reference In"=w311, "error in"=w312, "Number of Elements"=u32 512, "Timeout (ms)"=-1) -> ("FPGA VI Reference Out"=w308:refnum<k20>, "error out"=w309:errorcluster, "Data"=w314:fxp<+,44,44>[])  [unwired: 1 out]
            n76 = To Double Precision Float(number=w314) -> (double precision float=w313:dbl[])
            n77 = Square Root(x=w313) -> (sqrt(x)=w306:dbl[])
            n78 = Split 1D Array(array=w306, index=256) -> (first subarray=w304:dbl[], second subarray=w303:dbl[])
            "First FFT (bin)" <- w304
            "Second FFT (bin)" <- w303
            n79 = xnode "Invoke Method"("FPGA VI Reference In"=w308, "error in"=w309, "Number of Elements"=u32 0) -> ("error out"=w310:errorcluster)  [unwired: 1 in, 3 out]
            n80 = call "Distance-Velocity Calculation RT.vi"("First FFT"=w304, "Second FFT"=w303, "Windowing"=w294, "first FFT bin"=w297, "Sample Rate (S/s)"=w292, "last FFT bin"=w298) -> ("F_rise"=→"f_rise":dbl, "maxbin_firstFFT"=→"maxbin_firstFFT":i32, "maxbin_secondFFT"=→"maxbin_secondFFT":i32, "Distance (m)"=→"Distance (m)":dbl, "f_mean"=→"f_mean":dbl, "F_fall"=→"f_fall":dbl, "Velocity (m/s)"=→"Velocity (m/s)":dbl)  [unwired: 7 in]
          }
        }
      }
      frame #2 {
        n81 = case shown="True" w321 {
          tunnel: w318 -> [w324 w328]
          tunnel: [w324 w329] -> w317
          frame False {
          }
          frame True {
            n82 = Decrement(x="tieni premuto per") -> (x-1=w325:i32)
            n83 = Greater Or Equal?(x=w328, y=w325) -> (x >= y?=w327:bool)
            n84 = case shown="True" w327 {
              tunnel: w328 -> [w330 _]
              tunnel: [w331 0] -> w329
              frame False {
                n85 = Increment(x=w330) -> (x+1=w331:i32)
              }
              frame True {
                n86 = local write "Snapshot"(FALSE ("Snapshot")) -> ()
              }
            }
          }
        }
      }
    }
    n87 = node-c288() -> ()  [unwired: 1 in, 1 out]
  }
  n88 = node-c288(w41) -> ()  [unwired: 1 out]
  n89 = RT FIFO Delete(0:w21, 3:w20) -> (11:w19:errorcluster)  [unwired: 1 in]
  n90 = Merge Errors(w38, w39, w24, w19) -> (w22:errorcluster)
  n91 = flat-sequence {
    tunnel: w22 -> [w337]
    tunnel: w33 -> [w334]
    frame #0 {
      n92 = property class="Bool (strict)"(error in=w337, "Value"=FALSE ("stop")) -> (error out=w336:errorcluster)  [unwired: 1 in, 1 out]
      n93 = xnode "Invoke Method"("FPGA VI Reference In"=w334, "error in"=w336) -> ("FPGA VI Reference Out"=w339:refnum<k20>, "error out"=w338:errorcluster)
      n94 = xnode "Invoke Method"("FPGA VI Reference In"=w339, "error in"=w338) -> ("FPGA VI Reference Out"=w340:refnum<k20>, "error out"=w341:errorcluster)
      n95 = xnode "Close FPGA VI Reference"("FPGA VI Reference In"=w340, "error in"=w341) -> ()  [unwired: 1 out]
    }
  }
